vi "patientTrainingDetailView.vi"() -> ()   [LabVIEW 2019]
doc: "40"
uses:
  03_Home/controller/logoutBtn.ctl
  03_Home/controller/exitBtn.ctl
  <vilib>/Utility/miscctls.llb/LVPointTypeDef.ctl
  subVI/patients_state.ctl
  03_Home/controller/pannelState.ctl
  globalValue.vi
panel:
  out "training_duration":string
  out "assistance_level":string
  out "start_time":string
  out "exercise_date":string
  in  "back":bool
  in  "download":bool
  in  "backPage":bool
  out "training_id":string[](array[string])
  out "totalCount":string
  out "patients_nm":string
  out "patients_id":string
  in  "patients_weight":dbl format="%.1f kg"
  in  "patients_age":dbl
  in  "patients_height":dbl format="%.1f cm"
  out "patients_birthdate":dbl format="%<%Y.%m.%d.>T"
  in  "btnGroup":T1
  out "totalPage":i8
  out "crrentPage":i8
  in  "leftBtn":bool
  in  "rightBtn":bool
  in  "patientList":i32(listbox)
  out "userDetailInfo":string[](array[string])
  in  "Help Button":bool
  in  "LogOut Button":T2
  in  "Exit Button":T3
  out "userNm":string
  # "/"
  # "|"
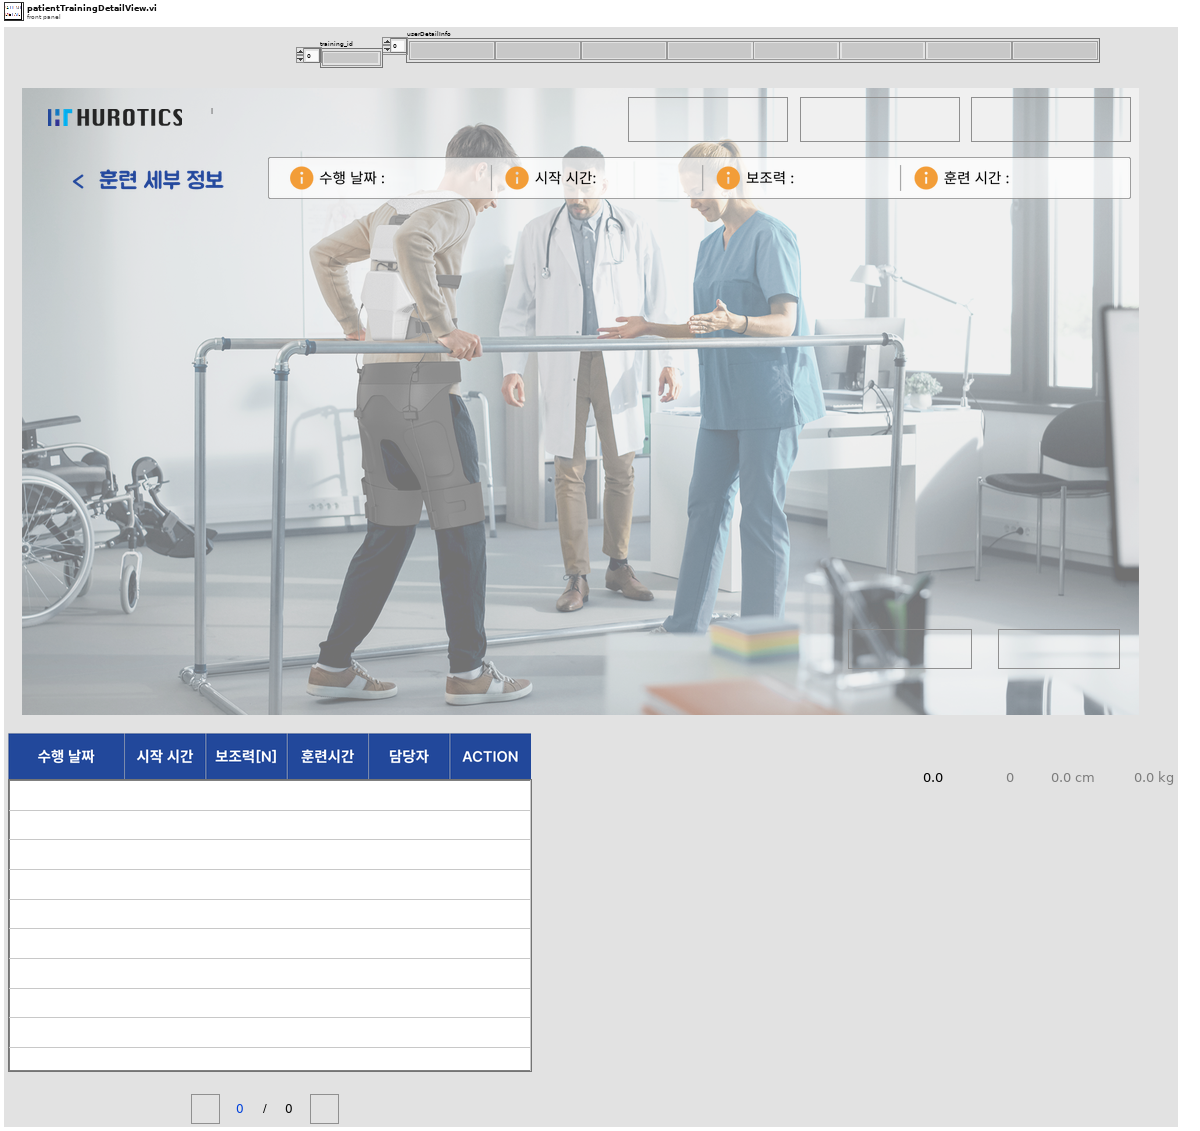
[diagram p1: front panel]
types:
  T1 = cluster{"detailBtn":bool, "detailBtn":bool, "detailBtn 2":bool, "detailBtn 3":bool, "detailBtn 4":bool, "detailBtn 5":bool, "detailBtn 6":bool, "detailBtn 7":bool, "detailBtn 8":bool, "detailBtn 9":bool}
  T2 = typedef "logoutBtn.ctl" = bool
  T3 = typedef "exitBtn.ctl" = bool
  T4 = typedef "LVPointTypeDef.ctl" = cluster{"Horizontal":i16, "Vertical":i16}
  T5 = typedef "patients_state.ctl" = enum16{"connection", "create", "getReadList", "getRead", "getCount", "update", "delete", "trash", "restore", "close"}
  T6 = enum16{"connection", "create", "getReadList", "getRead", "getCount", "update", "delete", "close"}
  T7 = enum8{"Enabled", "Disabled", "Disabled and Grayed Out"}
  T8 = typedef "pannelState.ctl" = enum16{"Init", "LogIn", "SignUpView", "Home", "Management_patientList", "Management_patientTrashtList", "Management_patientCreate", "Management_patientUpdate", "Management_patientTraining", "Management_patientTrainingDetail", "H-MEDI PatientList", "H-MEDI HardwareCtl", "Adjust", "FineTuning", "UserList", "UserDetail", "Exit"}
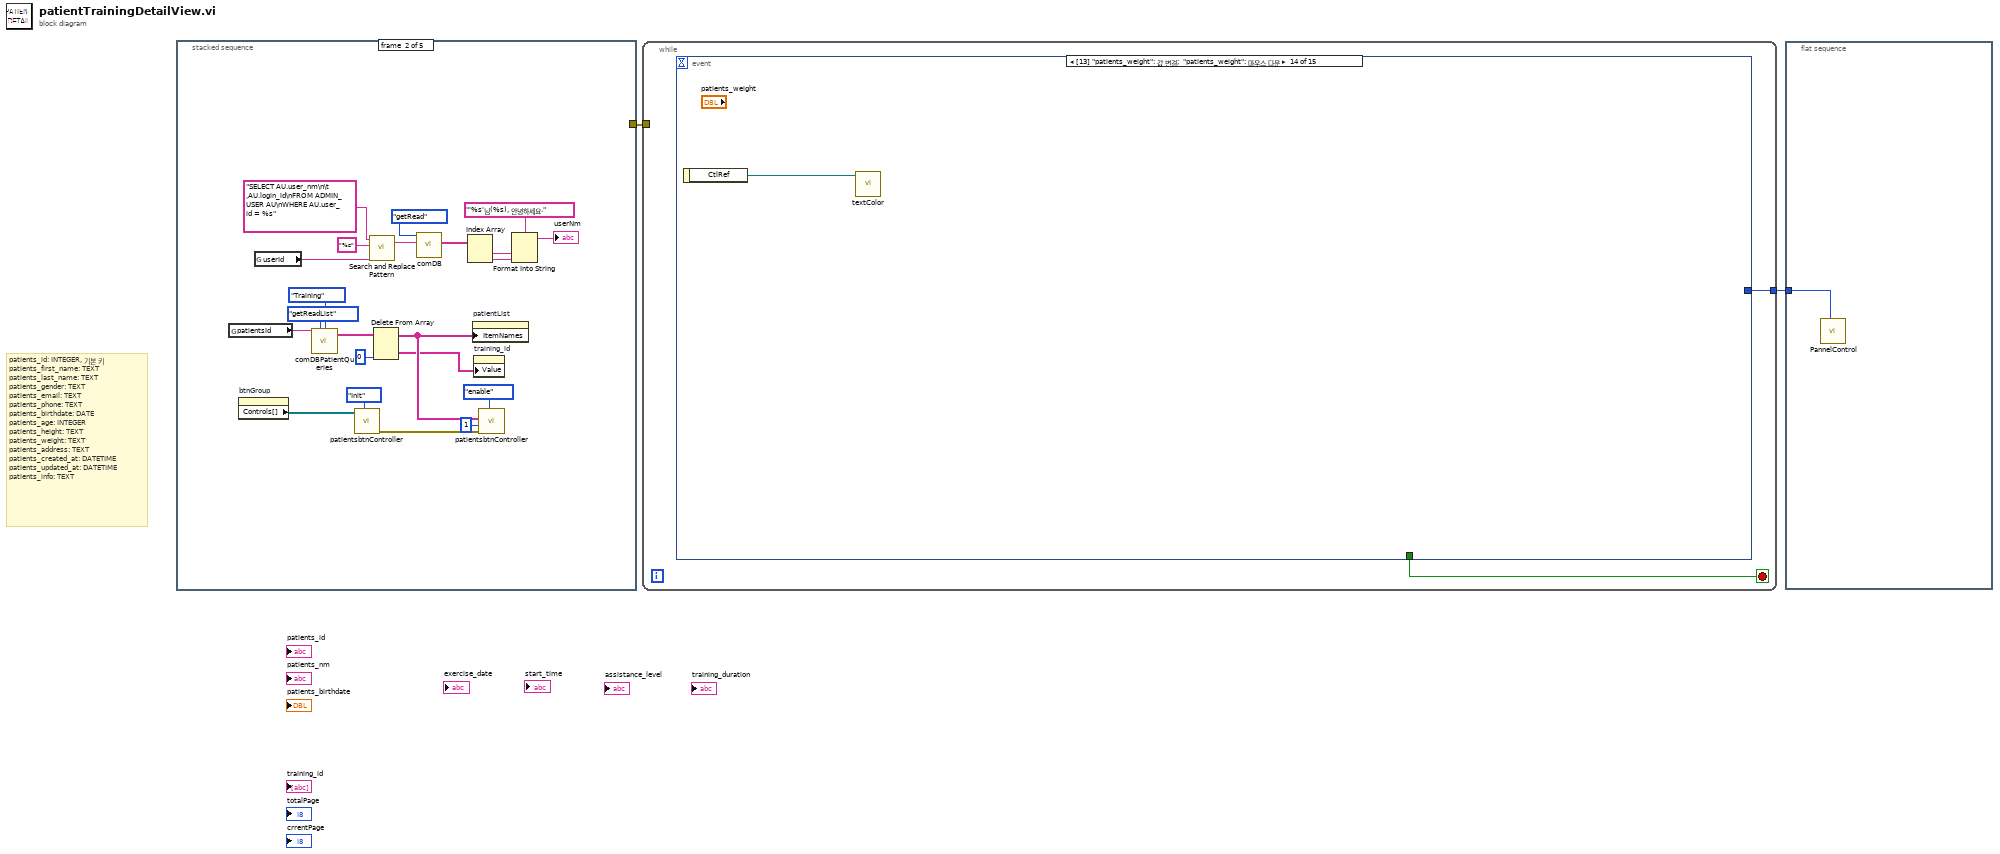
[diagram p0: block diagram]
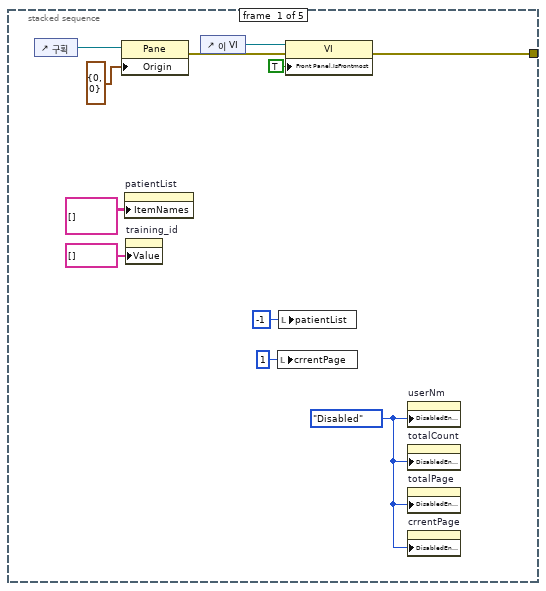
[diagram p2: hidden frame]
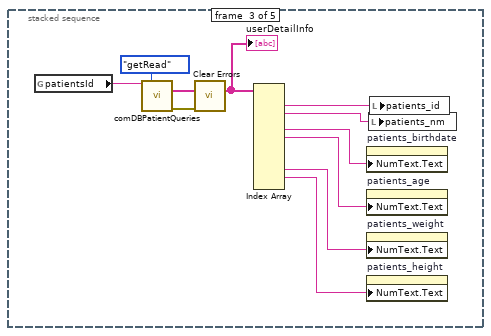
[diagram p3: hidden frame]
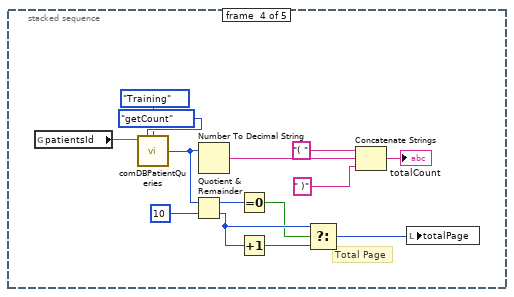
[diagram p4: hidden frame]
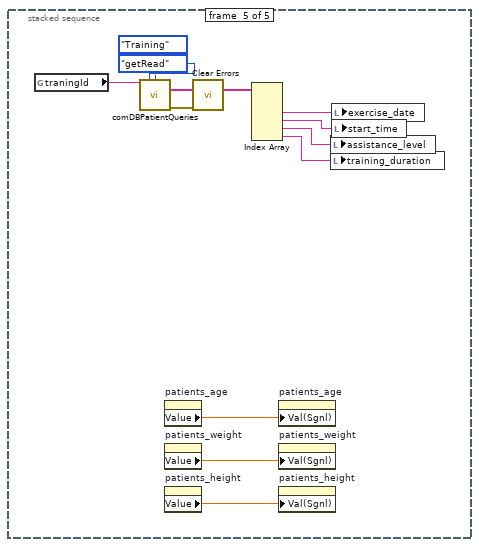
[diagram p5: hidden frame]
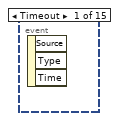
[diagram p6: hidden frame]
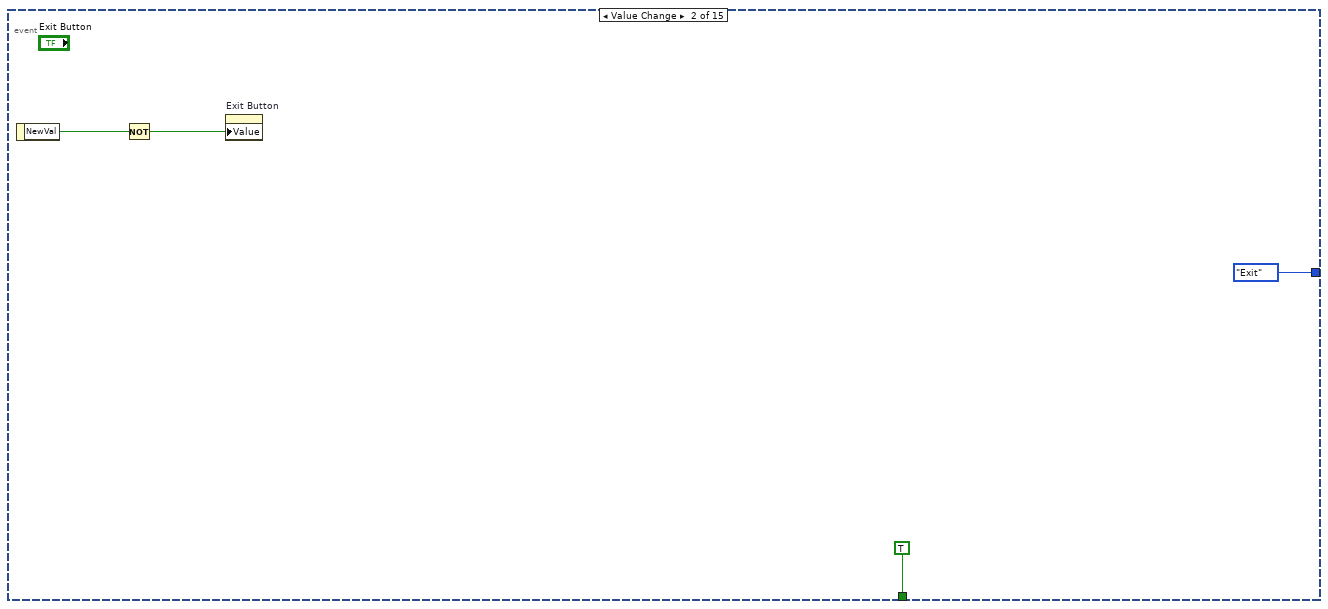
[diagram p7: hidden frame]
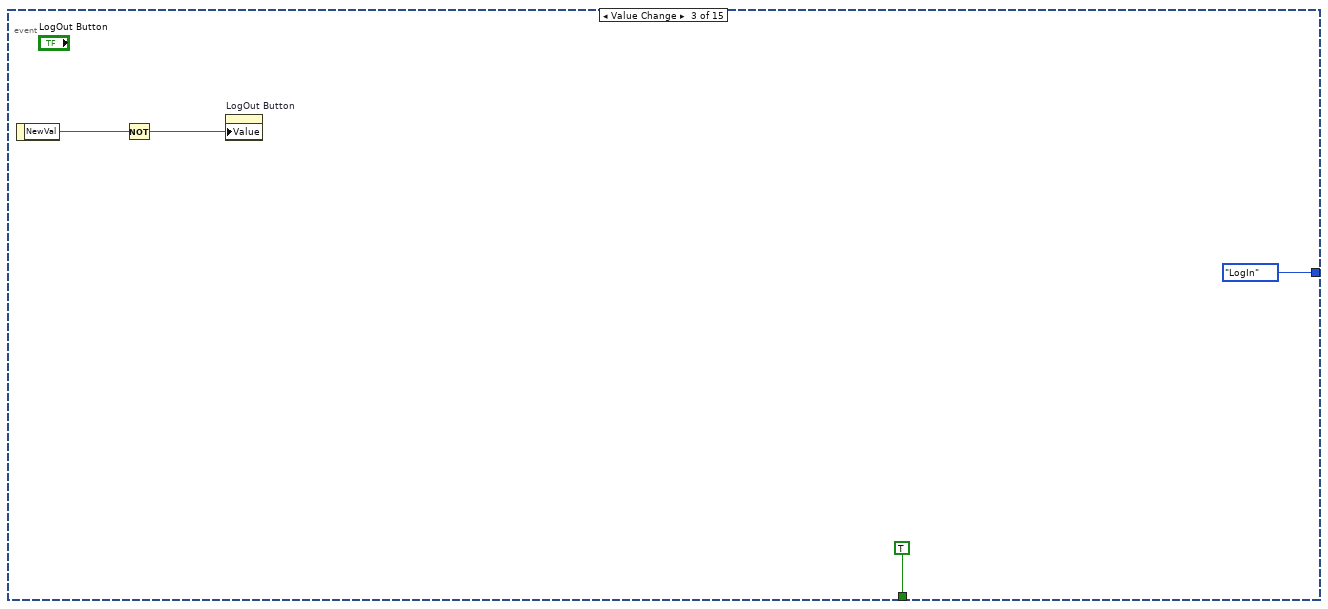
[diagram p8: hidden frame]
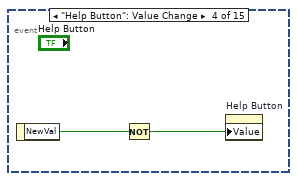
[diagram p9: hidden frame]
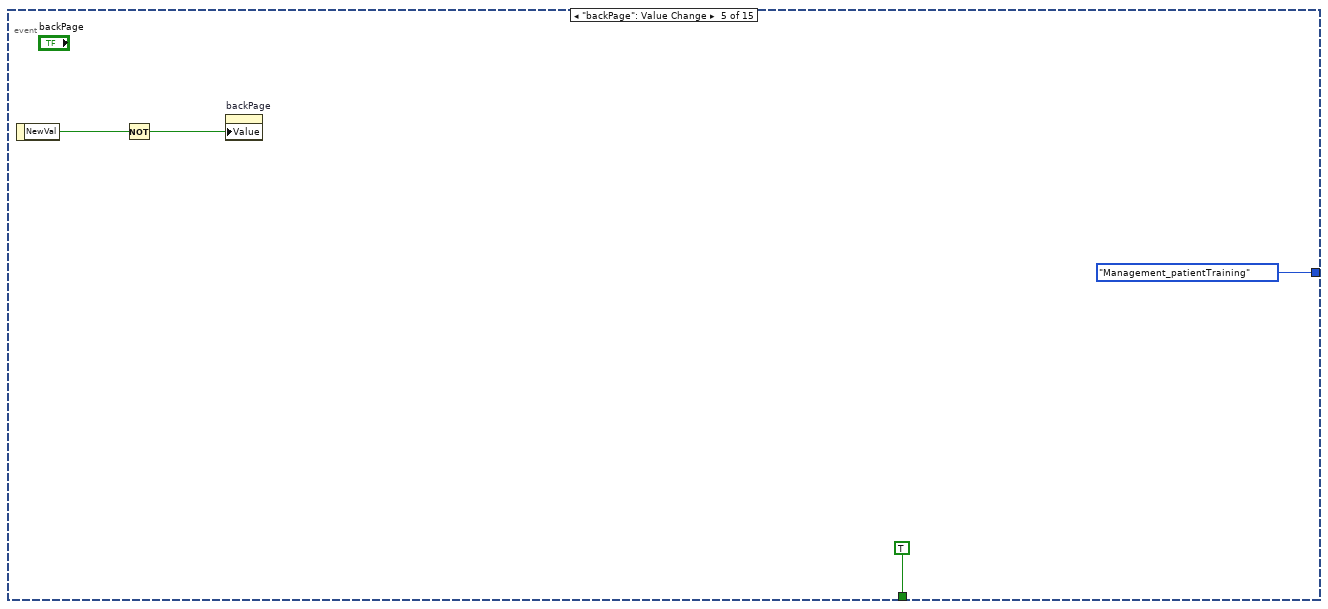
[diagram p10: hidden frame]
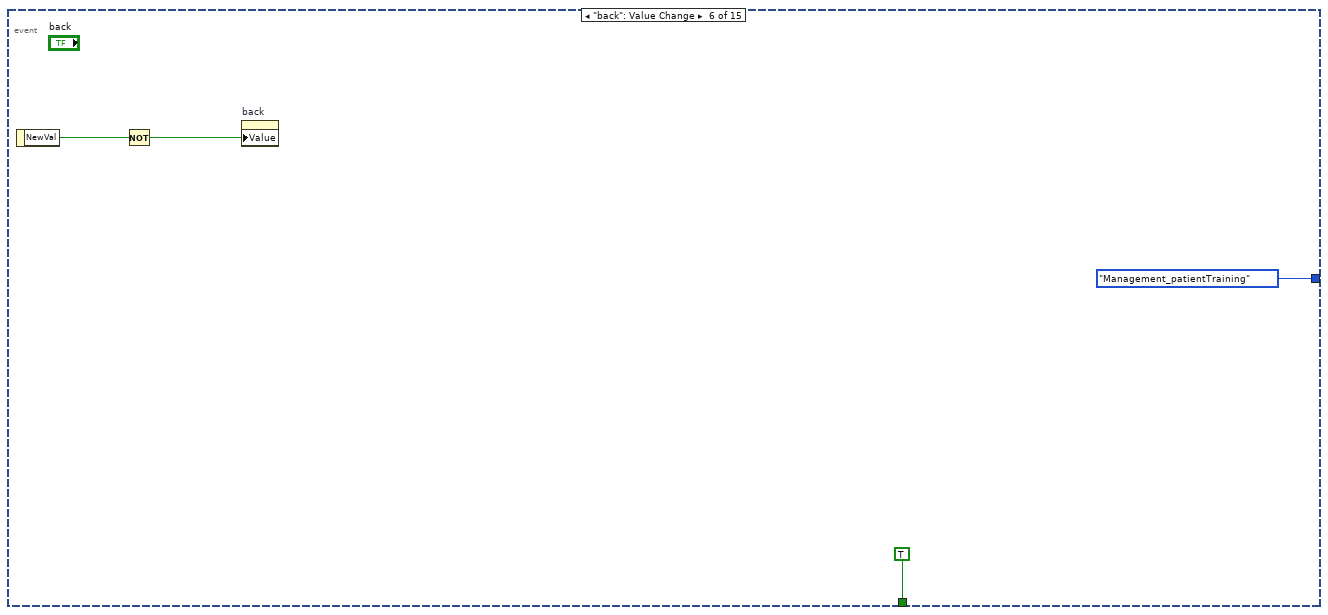
[diagram p11: hidden frame]
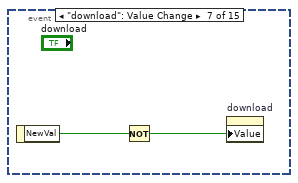
[diagram p12: hidden frame]
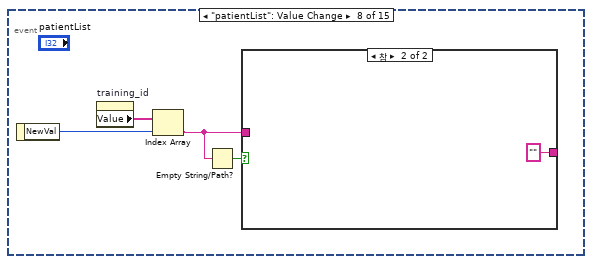
[diagram p13: hidden frame]
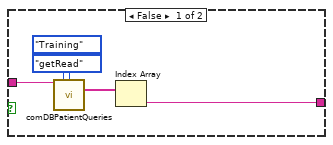
[diagram p14: hidden frame]
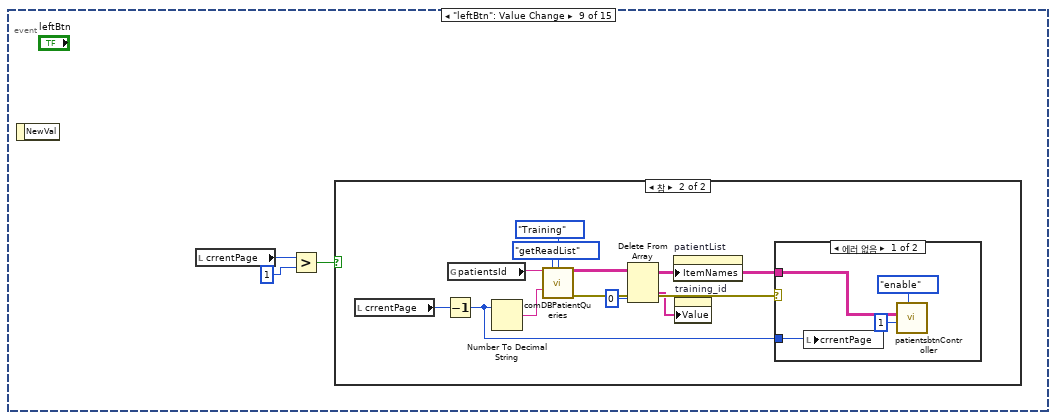
[diagram p15: hidden frame]
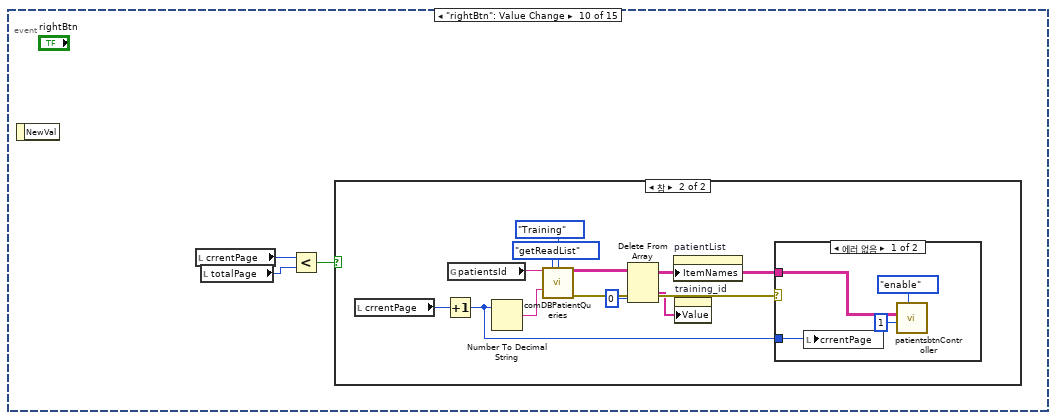
[diagram p18: hidden frame]
diagram:
  # "patients_id: INTEGER, 기본 키\npatients_first_name: TEXT\npatients_last_name: TEXT\npatients_gender: TEXT\npatients_email: TEXT\npatients_phone: TEXT\npatients_birthdate: DATE\npatients_age: INTEGER\npatients_height: TEXT\npatients_weight: TEXT\npatients_address: TEXT\npatients_created_at: DATETIME\npatients_updated_at: DATETIME\npatients_info: TEXT"
  n1 = stacked-sequence {
    tunnel: [w8 _ _ _ _] -> w1
    frame #0 {
      w6 = T7."Disabled" ("비활성화")
      n2 = control-ref of="구획"() -> (w11:refnum<vi>)
      n3 = property class="Pane"(reference=w11, "Origin"=T4 {"Horizontal"=0, "Vertical"=0} ("원점")) -> (error out=w9:errorcluster)  [unwired: 1 in, 1 out]
      n4 = property on="patientList" class="MCListbox (엄격한)"("ItemNames"=string[][] [] ("아이템 이름")) -> ()  [unwired: 2 in, 2 out]
      n5 = property on="training_id" class="Arr (엄격한)"("Value"=string[] [] ("training_id")) -> ()  [unwired: 2 in, 2 out]
      n6 = control-ref of="이 VI"() -> (w13:refnum<vi>)
      n7 = local write "crrentPage"(i8 1 ("crrentPage")) -> ()
      n8 = local write "patientList"(-1 ("patientList")) -> ()
      n9 = property class="VI"(reference=w13, error in=w9, "Front Panel.IsFrontmost"=TRUE ("프런트패널 윈도우:맨 앞으로")) -> (error out=w8:errorcluster)  [unwired: 1 out]
      n10 = property on="userNm" class="Str"("DisabledEnum"=w6) -> ()  [unwired: 2 in, 2 out]
      n11 = property on="totalCount" class="Str"("DisabledEnum"=w6) -> ()  [unwired: 2 in, 2 out]
      n12 = property on="totalPage" class="DigNum (엄격한)"("DisabledEnum"=w6) -> ()  [unwired: 2 in, 2 out]
      n13 = property on="crrentPage" class="DigNum (엄격한)"("DisabledEnum"=w6) -> ()  [unwired: 2 in, 2 out]
    }
    frame #1 {
      n14 = global read "globalValue.vi" "patientsId"() -> (w15:string)
      n15 = property on="btnGroup" class="Clust"() -> ("Controls[]"=w20:refnum<vi>[])  [unwired: 2 in, 2 out]
      n16 = global read "globalValue.vi" "userId"() -> (w26:string)
      n17 = call "comDBPatientQueries.vi"("id"=w15, "State"=patients_state."getReadList", "select"=enum16{"Default", "Trash", "Training"}."Training") -> ("resultList"=w19:string[][])  [unwired: 9 in, 3 out]
      n18 = call "patientsbtnController.vi"("state"=enum16{"Init", "disable", "enable"}."Init", "Controls[]"=w20) -> ("error out"=w24:errorcluster)  [unwired: 9 in]
      n19 = call <vilib>:"Search and Replace Pattern.vi"("string"="SELECT AU.user_nm\n\t         ,AU.login_id\nFROM ADMIN_USER AU\nWHERE AU.user_id = %s" ("Query"), "regular expression (\"\")"="%s" ("regular expression (\"\")"), "replace string (\"\")"=w26) -> ("result string"=w27:string)  [unwired: 2 in, 1 out]
      n20 = Delete From Array(array=w19, index (col)=0 ("비활성화된 인덱스 (열)")) -> (deleted portion=w16:string[], array with subset deleted=w17:string[][])  [unwired: 2 in]
      n21 = call "comDB.vi"("Query"=w27, "State"=T6."getRead") -> ("result1DArray"=w33:string[])  [unwired: 5 in, 3 out]
      n22 = Index Array(array=w33) -> (element #1=w32:string, element #2=w31:string)  [unwired: 2 in]
      n23 = property on="patientList" class="MCListbox (엄격한)"("ItemNames"=w17) -> ()  [unwired: 2 in, 2 out]
      n24 = property on="training_id" class="Arr (엄격한)"("Value"=w16) -> ()  [unwired: 2 in, 2 out]
      n25 = call "patientsbtnController.vi"("state"=enum16{"Init", "disable", "enable"}."enable", "error in (no error)"=w24, "버튼개수"=1, "2dArray"=w17) -> ()  [unwired: 7 in, 1 out]
      n26 = Format Into String(format string="'%s'님(%s), 안녕하세요." ("문자열"), w32, w31) -> (resulting string=→"userNm":string)  [unwired: 2 in, 1 out]
    }
    frame #2 {
      n27 = global read "globalValue.vi" "patientsId"() -> (w40:string)
      n28 = call "comDBPatientQueries.vi"("id"=w40, "State"=patients_state."getRead") -> ("result1DArray"=w45:string[], "error out"=w44:errorcluster)  [unwired: 10 in, 2 out]
      "userDetailInfo" <- w45
      n29 = call <vilib>:"Clear Errors.vi"("error in (no error)"=w44) -> ()  [unwired: 5 in, 2 out]
      n30 = Index Array(array=w45) -> (element #1=w42:string, element #2=w41:string, element #4=w39:string, element #5=w38:string, element #9=w37:string, element #10=w36:string)  [unwired: 11 in, 5 out]
      n31 = property on="patients_birthdate" class="DigNum (엄격한)"("NumText.Text"=w39) -> ()  [unwired: 2 in, 2 out]
      n32 = property on="patients_age" class="DigNum (엄격한)"("NumText.Text"=w38) -> ()  [unwired: 2 in, 2 out]
      n33 = property on="patients_weight" class="DigNum (엄격한)"("NumText.Text"=w37) -> ()  [unwired: 2 in, 2 out]
      n34 = property on="patients_height" class="DigNum (엄격한)"("NumText.Text"=w36) -> ()  [unwired: 2 in, 2 out]
      n35 = local write "patients_nm"(w41) -> ()
      n36 = local write "patients_id"(w42) -> ()
    }
    frame #3 {
      # "Total Page"
      n37 = global read "globalValue.vi" "patientsId"() -> (w46:string)
      n38 = call "comDBPatientQueries.vi"("id"=w46, "State"=patients_state."getCount", "select"=enum16{"Default", "Trash", "Training"}."Training") -> ("count"=w59:i64)  [unwired: 9 in, 3 out]
      n39 = Quotient & Remainder(x=w59, y=i64 10) -> (x-y*floor(x/y)=w57:i64, floor(x/y)=w58:i64)
      n40 = Number To Decimal String(number=w59) -> (decimal integer string=w53:string)  [unwired: 1 in]
      n41 = Equal To 0?(x=w57) -> (x = 0?=w56:bool)
      n42 = Increment(x=w58) -> (x+1=w55:i64)
      n43 = Select(t=w58, s=w56, f=w55) -> (s? t:f=w48:i64)
      n44 = Concatenate Strings("( ", w53, " )") -> (→"totalCount":string)
      n45 = local write "totalPage"(w48) -> ()
    }
    frame #4 {
      n46 = global read "globalValue.vi" "traningId"() -> (w66:string)
      n47 = call "comDBPatientQueries.vi"("id"=w66, "State"=patients_state."getRead", "select"=enum16{"Default", "Trash", "Training"}."Training") -> ("result1DArray"=w68:string[], "error out"=w67:errorcluster)  [unwired: 9 in, 2 out]
      n48 = property on="patients_age" class="DigNum (엄격한)"() -> ("Value"=w71:dbl)  [unwired: 2 in, 2 out]
      n49 = property on="patients_weight" class="DigNum (엄격한)"() -> ("Value"=w70:dbl)  [unwired: 2 in, 2 out]
      n50 = property on="patients_height" class="DigNum (엄격한)"() -> ("Value"=w69:dbl)  [unwired: 2 in, 2 out]
      n51 = call <vilib>:"Clear Errors.vi"("error in (no error)"=w67) -> ()  [unwired: 5 in, 2 out]
      n52 = Index Array(array=w68) -> (element #2=w63:string, element #3=w62:string, element #4=w61:string, element #5=w60:string)  [unwired: 5 in, 1 out]
      n53 = property on="patients_age" class="DigNum (엄격한)"("Val(Sgnl)"=w71) -> ()  [unwired: 2 in, 2 out]
      n54 = property on="patients_weight" class="DigNum (엄격한)"("Val(Sgnl)"=w70) -> ()  [unwired: 2 in, 2 out]
      n55 = property on="patients_height" class="DigNum (엄격한)"("Val(Sgnl)"=w69) -> ()  [unwired: 2 in, 2 out]
      n56 = local write "assistance_level"(w61) -> ()
      n57 = local write "training_duration"(w60) -> ()
      n58 = local write "exercise_date"(w63) -> ()
      n59 = local write "start_time"(w62) -> ()
    }
  }
  n60 = while {
    tunnel: [w72] -> w2
    tunnel: w1 -> [_]
    stop <- w73 stop-if-true
    n61 = event shown="[13] \"patients_weight\": 값 변경;  \"patients_weight\": 마우스 다운" {
      selector: _ -> [_ _ _ _ _ _ _ _ _ _ _ _ _ _ _]
      dyn-events: _ -> [_ _ _ _ _ _ _ _ _ _ _ _ _ _ _]
      timeout: _ -> [_ _ _ _ _ _ _ _ _ _ _ _ _ _ _]
      tunnel: [_ TRUE TRUE _ TRUE TRUE _ _ _ _ TRUE w149 _ _ _] -> w73
      tunnel: [_ pannelState."Exit" ("State") pannelState."LogIn" ("State") _ pannelState."Management_patientTraining" ("State") pannelState."Management_patientTraining" ("State") _ _ _ _ pannelState."Management_patientTrainingDetail" ("State") pannelState."Management_patientTrainingDetail" ("State") _ _ _] -> w72
      event Timeout {
        n62 = event-data() -> ()  [unwired: 1 in, 3 out]
      }
      event Value Change {
        n63 = event-data() -> ("NewVal"=w75:T3)  [unwired: 1 in]
        n64 = Not(x=w75) -> (.not. x?=w74:T3)
        n65 = property on="Exit Button" class="Bool (엄격한)"("Value"=w74) -> ()  [unwired: 2 in, 2 out]
      }
      event Value Change {
        n66 = event-data() -> ("NewVal"=w79:T2)  [unwired: 1 in]
        n67 = Not(x=w79) -> (.not. x?=w78:T2)
        n68 = property on="LogOut Button" class="Bool (엄격한)"("Value"=w78) -> ()  [unwired: 2 in, 2 out]
      }
      event "Help Button": Value Change {
        n69 = event-data() -> ("NewVal"=w83:bool)  [unwired: 1 in]
        n70 = Not(x=w83) -> (.not. x?=w82:bool)
        n71 = property on="Help Button" class="Bool (엄격한)"("Value"=w82) -> ()  [unwired: 2 in, 2 out]
      }
      event "backPage": Value Change {
        n72 = event-data() -> ("NewVal"=w86:bool)  [unwired: 1 in]
        n73 = Not(x=w86) -> (.not. x?=w85:bool)
        n74 = property on="backPage" class="Bool (엄격한)"("Value"=w85) -> ()  [unwired: 2 in, 2 out]
      }
      event "back": Value Change {
        n75 = event-data() -> ("NewVal"=w91:bool)  [unwired: 1 in]
        n76 = Not(x=w91) -> (.not. x?=w88:bool)
        n77 = property on="back" class="Bool (엄격한)"("Value"=w88) -> ()  [unwired: 2 in, 2 out]
      }
      event "download": Value Change {
        n78 = event-data() -> ("NewVal"=w93:bool)  [unwired: 1 in]
        n79 = Not(x=w93) -> (.not. x?=w92:bool)
        n80 = property on="download" class="Bool (엄격한)"("Value"=w92) -> ()  [unwired: 2 in, 2 out]
      }
      event "patientList": Value Change {
        n81 = event-data() -> ("NewVal"=w96:i32)  [unwired: 1 in]
        n82 = property on="training_id" class="Arr (엄격한)"() -> ("Value"=w97:string[])  [unwired: 2 in, 2 out]
        n83 = Index Array(array=w97, index=w96) -> (element=w95:string)
        n84 = Empty String/Path?(string/path=w95) -> (empty?=w94:bool)
        n85 = case shown="참" w94 {
          tunnel: w95 -> [w99 _]
          tunnel: [w98 "" ("Text")] -> _
          frame False {
            n86 = call "comDBPatientQueries.vi"("id"=w99, "State"=patients_state."getRead", "select"=enum16{"Default", "Trash", "Training"}."Training") -> ("result1DArray"=w100:string[])  [unwired: 9 in, 3 out]
            n87 = Index Array(array=w100) -> (element=w98:string)  [unwired: 1 in]
          }
          frame True {
          }
        }
      }
      event "leftBtn": Value Change {
        n88 = event-data() -> ()  [unwired: 1 in, 1 out]
        n89 = local read "crrentPage"() -> (w106:i8)
        n90 = Greater?(x=w106, y=1) -> (0:w105:bool)
        n91 = case shown="참" w105 {
          frame False {
          }
          frame True {
            n92 = local read "crrentPage"() -> (w113:i8)
            n93 = Decrement(x=w113) -> (x-1=w117:i8)
            n94 = global read "globalValue.vi" "patientsId"() -> (w107:string)
            n95 = Number To Decimal String(number=w117) -> (decimal integer string=w115:string)  [unwired: 1 in]
            n96 = call "comDBPatientQueries.vi"("id"=w107, "State"=patients_state."getReadList", "select"=enum16{"Default", "Trash", "Training"}."Training", "crrentPage"=w115) -> ("resultList"=w110:string[][], "error out"=w114:errorcluster)  [unwired: 8 in, 2 out]
            n97 = Delete From Array(array=w110, index (col)=0 ("비활성화된 인덱스 (열)")) -> (deleted portion=w108:string[], array with subset deleted=w109:string[][])  [unwired: 2 in]
            n98 = property on="patientList" class="MCListbox (엄격한)"("ItemNames"=w109) -> ()  [unwired: 2 in, 2 out]
            n99 = property on="training_id" class="Arr (엄격한)"("Value"=w108) -> ()  [unwired: 2 in, 2 out]
            n100 = case shown="에러 없음" w114 {
              tunnel: w117 -> [w119 _]
              tunnel: w109 -> [w120 _]
              frame No Error {
                n101 = local write "crrentPage"(w119) -> ()
                n102 = call "patientsbtnController.vi"("state"=enum16{"Init", "disable", "enable"}."enable", "버튼개수"=1, "2dArray"=w120) -> ()  [unwired: 8 in, 1 out]
              }
              frame Error {
              }
            }
          }
        }
      }
      event "rightBtn": Value Change {
        n103 = event-data() -> ()  [unwired: 1 in, 1 out]
        n104 = local read "crrentPage"() -> (w124:i8)
        n105 = local read "totalPage"() -> (w122:i8)
        n106 = Less?(x=w124, y=w122) -> (x < y?=w123:bool)
        n107 = case shown="참" w123 {
          frame False {
          }
          frame True {
            n108 = local read "crrentPage"() -> (w131:i8)
            n109 = Increment(x=w131) -> (x+1=w135:i8)
            n110 = global read "globalValue.vi" "patientsId"() -> (w125:string)
            n111 = Number To Decimal String(number=w135) -> (decimal integer string=w133:string)  [unwired: 1 in]
            n112 = call "comDBPatientQueries.vi"("id"=w125, "State"=patients_state."getReadList", "select"=enum16{"Default", "Trash", "Training"}."Training", "crrentPage"=w133) -> ("resultList"=w128:string[][], "error out"=w132:errorcluster)  [unwired: 8 in, 2 out]
            n113 = Delete From Array(array=w128, index (col)=0 ("비활성화된 인덱스 (열)")) -> (deleted portion=w126:string[], array with subset deleted=w127:string[][])  [unwired: 2 in]
            n114 = property on="patientList" class="MCListbox (엄격한)"("ItemNames"=w127) -> ()  [unwired: 2 in, 2 out]
            n115 = property on="training_id" class="Arr (엄격한)"("Value"=w126) -> ()  [unwired: 2 in, 2 out]
            n116 = case shown="에러 없음" w132 {
              tunnel: w135 -> [w137 _]
              tunnel: w127 -> [w138 _]
              frame No Error {
                n117 = local write "crrentPage"(w137) -> ()
                n118 = call "patientsbtnController.vi"("state"=enum16{"Init", "disable", "enable"}."enable", "버튼개수"=1, "2dArray"=w138) -> ()  [unwired: 8 in, 1 out]
              }
              frame Error {
              }
            }
          }
        }
      }
      event "btnGroup": Value Change {
        n119 = event-data() -> ("NewVal"=w145:T1)  [unwired: 1 in]
        n120 = Cluster To Array(cluster=w145) -> (array=w147:bool[])
        n121 = Search 1D Array(1D array=w147, element=TRUE ("원소")) -> (index of element=w144:i32)  [unwired: 1 in]
        n122 = property on="training_id" class="Arr (엄격한)"() -> ("Value"=w143:string[])  [unwired: 2 in, 2 out]
        n123 = Index Array(array=w143, index=w144) -> (element=w140:string)
        n124 = global write "globalValue.vi" "traningId"(w140) -> ()
      }
      event "patientList": Double Click {
        n125 = event-data() -> ("Row"=w152:i32)  [unwired: 1 in]
        n126 = property on="training_id" class="Arr (엄격한)"() -> ("Value"=w153:string[])  [unwired: 2 in, 2 out]
        n127 = Index Array(array=w153, index=w152) -> (element=w150:string)
        n128 = Empty String/Path?(string/path=w150) -> (empty?=w151:bool)
        n129 = case shown="거짓" w151 {
          tunnel: w150 -> [w155 _]
          tunnel: [TRUE _] -> w149
          frame False {
            n130 = global write "globalValue.vi" "traningId"(w155) -> ()
          }
          frame True {
          }
        }
      }
      event "patients_age": Value Change; "patients_age": Mouse Down {
        n131 = event-data() -> ("CtlRef"=w156:refnum<vi>)  [unwired: 1 in]
        n132 = call "textColor.vi"("디지털 입력"=w156) -> ()  [unwired: 11 in]
      }
      event "patients_weight": Value Change; "patients_weight": Mouse Down {
        n133 = event-data() -> ("CtlRef"=w157:refnum<vi>)  [unwired: 1 in]
        n134 = call "textColor.vi"("디지털 입력"=w157) -> ()  [unwired: 11 in]
      }
      event "patients_height": Value Change; "patients_height": Mouse Down {
        n135 = event-data() -> ("CtlRef"=w158:refnum<vi>)  [unwired: 1 in]
        n136 = call "textColor.vi"("디지털 입력"=w158) -> ()  [unwired: 11 in]
      }
    }
  }
  n137 = flat-sequence {
    tunnel: w2 -> [w159]
    frame #0 {
      n138 = call "PannelControl.vi"("State"=w159) -> ()  [unwired: 10 in, 1 out]
    }
  }
